vi "HHSetResol.vi"(2 "DeviceIndex":i32, 4 "Binning":i32 min=0 max=5 step=1) -> (0 "Resolution":dbl format="%.2f", 1 "error":i32)   [LabVIEW 2009]
uses:
  hhlib.dll
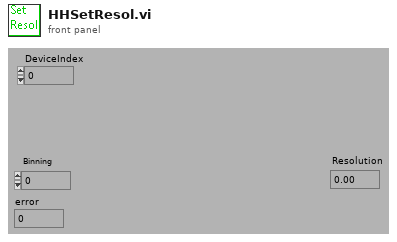
[diagram p1: front panel]
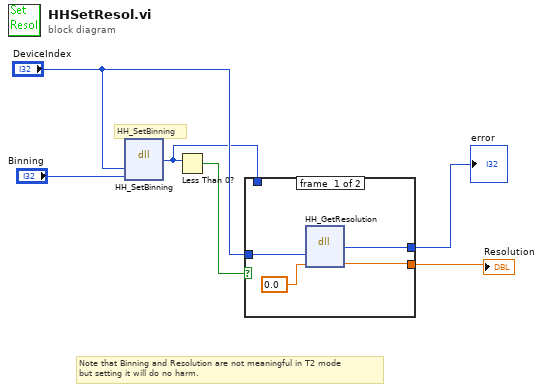
[diagram p0: block diagram]
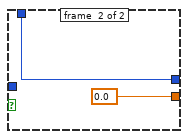
[diagram p2: hidden frame]
diagram:
  # "HH_SetBinning"
  # "Note that Binning and Resolution are not meaningful in T2 mode\nbut setting it will do no harm."
  n1 = dll-call lib="C:/Programme/Anwendungen/DAQLinescan_HH/hhlib.dll" fn="HH_SetBinning"("devidx"="DeviceIndex", "Range"="Binning") -> (w2:i32)  [unwired: 5 in, 2 out]
  n2 = Less Than 0?(x=w2) -> (x < 0?=w3:bool)
  n3 = case shown="False" w3 {
    tunnel: [w8 0.0] -> w4
    tunnel: "DeviceIndex" -> [w10 _]
    tunnel: [w7 w11] -> w1
    tunnel: w2 -> [_ w11]
    frame #0 {
      n4 = dll-call lib="C:/Programme/Anwendungen/DAQLinescan_HH/hhlib.dll" fn="HH_GetResolution"("devidx"=w10, "resolution"=0.0) -> (w7:i32, "resolution"=w8:dbl)  [unwired: 4 in, 2 out]
    }
    frame #1 {
    }
  }
  "Resolution" <- w4
  "error" <- w1
